vi "Clock Value.vi"() -> ()   [LabVIEW 2020]
panel:
  out "D 4":bool
  out "E 4":bool
  out "C 4":bool
  out "A 4":bool
  out "G 4":bool
  out "F 4":bool
  out "B 4":bool
  out "D 3":bool
  out "E 3":bool
  out "C 3":bool
  out "A 3":bool
  out "G 3":bool
  out "F 3":bool
  out "B 3":bool
  out "D 2":bool
  out "E 2":bool
  out "C 2":bool
  out "A 2":bool
  out "G 2":bool
  out "F 2":bool
  out "B 2":bool
  out "D":bool
  out "E":bool
  out "C":bool
  out "A":bool
  out "G":bool
  out "F":bool
  out "B":bool
  out "sig":bool
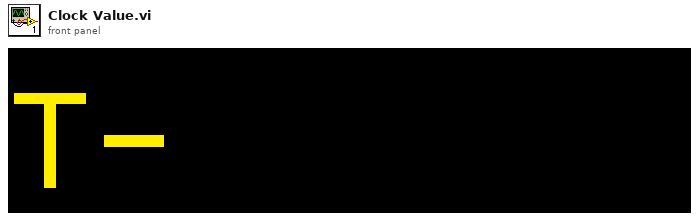
[diagram p1: front panel]
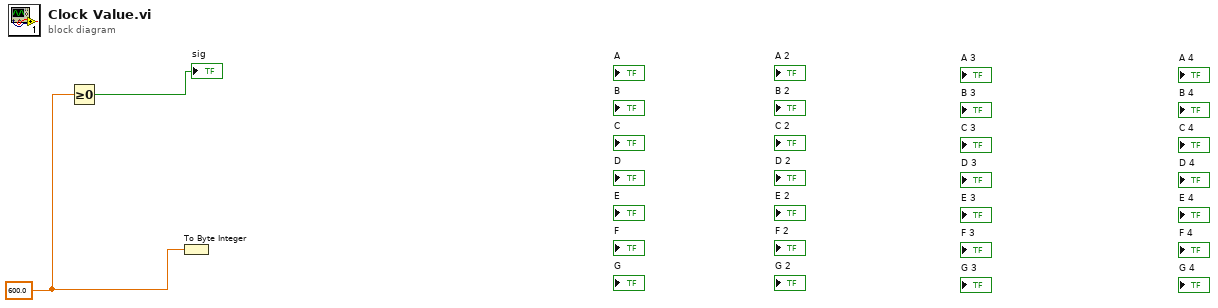
[diagram p0: block diagram]
diagram:
  w1 = 600.0
  n1 = Greater Or Equal To 0?(x=w1) -> (x >= 0?=→"sig":bool)
  n2 = To Byte Integer(number=w1) -> ()  [unwired: 1 out]
